vi "Add_spot_dialog.vi"(7 "Modify":bool, 8 "TransformedPt":bool, 9 "ArrayOfPointNames":string[](array[string]), 10 "CurrentSessionInformation_IN":T2={"CollectionOfPoints"=[{"MetaDataFile"=path "", "X"=0.0, "Y"=0.0, "Z"=0.0, "Group"=0, "Rotation"=0.0, "Fiducial"=FALSE, "Magnification"=0.0, "Working_Distance"=0.0, "Notes"="", "Location Name/ID"="", "OtherRelatedDataFiles"=[], "Available"=FALSE}, {"MetaDataFile"=path "", "X"=0.0, "Y"=0.0, "Z"=0.0, "Group"=0, "Rotation"=0.0, "Fiducial"=FALSE, "Magnification"=0.0, "Working_Distance"=0.0, "Notes"="", "Location Name/ID"="", "OtherRelatedDataFiles"=[], "Available"=FALSE}, {"MetaDataFile"=path "", "X"=0.0, "Y"=0.0, "Z"=0.0, "Group"=0, "Rotation"=0.0, "Fiducial"=FALSE, "Magnification"=0.0, "Working_Distance"=0.0, "Notes"="", "Location Name/ID"="", "OtherRelatedDataFiles"=[], "Available"=FALSE}, {"MetaDataFile"=path "", "X"=0.0, "Y"=0.0, "Z"=0.0, "Group"=0, "Rotation"=0.0, "Fiducial"=FALSE, "Magnification"=0.0, "Working_Distance"=0.0, "Notes"="", "Location Name/ID"="", "OtherRelatedDataFiles"=[], "Available"=FALSE}, {"MetaDataFile"=path "", "X"=0.0, "Y"=0.0, "Z"=0.0, "Group"=0, "Rotation"=0.0, "Fiducial"=FALSE, "Magnification"=0.0, "Working_Distance"=0.0, "Notes"="", "Location Name/ID"="", "OtherRelatedDataFiles"=[], "Available"=FALSE}, {"MetaDataFile"=path "", "X"=0.0, "Y"=0.0, "Z"=0.0, "Group"=0, "Rotation"=0.0, "Fiducial"=FALSE, "Magnification"=0.0, "Working_Distance"=0.0, "Notes"="", "Location Name/ID"="", "OtherRelatedDataFiles"=[], "Available"=FALSE}, {"MetaDataFile"=path "", "X"=0.0, "Y"=0.0, "Z"=0.0, "Group"=0, "Rotation"=0.0, "Fiducial"=FALSE, "Magnification"=0.0, "Working_Distance"=0.0, "Notes"="", "Location Name/ID"="", "OtherRelatedDataFiles"=[], "Available"=FALSE}], "Instrument"=enum."MXRD MFC", "CollectionFile"=path "/INL Macintosh/Users/timothymcjunkin/Desktop/Diffusion couple/MXRD 9-13-10/xrd_session_for_corrected.xml", "Session Name/ID"="xrd_test", "SessionNotes"="Sample moved to XRD"}, 11 "PointInformation_IN":T1) -> (0 "PointInformationOut":T1, 1 "CurrentSessionInformationOut":T2={"CollectionOfPoints"=[{"MetaDataFile"=path "", "X"=0.0, "Y"=0.0, "Z"=0.0, "Group"=0, "Rotation"=0.0, "Fiducial"=FALSE, "Magnification"=0.0, "Working_Distance"=0.0, "Notes"="", "Location Name/ID"="", "OtherRelatedDataFiles"=[], "Available"=FALSE}, {"MetaDataFile"=path "", "X"=0.0, "Y"=0.0, "Z"=0.0, "Group"=0, "Rotation"=0.0, "Fiducial"=FALSE, "Magnification"=0.0, "Working_Distance"=0.0, "Notes"="", "Location Name/ID"="", "OtherRelatedDataFiles"=[], "Available"=FALSE}, {"MetaDataFile"=path "", "X"=0.0, "Y"=0.0, "Z"=0.0, "Group"=0, "Rotation"=0.0, "Fiducial"=FALSE, "Magnification"=0.0, "Working_Distance"=0.0, "Notes"="", "Location Name/ID"="", "OtherRelatedDataFiles"=[], "Available"=FALSE}, {"MetaDataFile"=path "", "X"=0.0, "Y"=0.0, "Z"=0.0, "Group"=0, "Rotation"=0.0, "Fiducial"=FALSE, "Magnification"=0.0, "Working_Distance"=0.0, "Notes"="", "Location Name/ID"="", "OtherRelatedDataFiles"=[], "Available"=FALSE}, {"MetaDataFile"=path "", "X"=0.0, "Y"=0.0, "Z"=0.0, "Group"=0, "Rotation"=0.0, "Fiducial"=FALSE, "Magnification"=0.0, "Working_Distance"=0.0, "Notes"="", "Location Name/ID"="", "OtherRelatedDataFiles"=[], "Available"=FALSE}, {"MetaDataFile"=path "", "X"=0.0, "Y"=0.0, "Z"=0.0, "Group"=0, "Rotation"=0.0, "Fiducial"=FALSE, "Magnification"=0.0, "Working_Distance"=0.0, "Notes"="", "Location Name/ID"="", "OtherRelatedDataFiles"=[], "Available"=FALSE}, {"MetaDataFile"=path "", "X"=0.0, "Y"=0.0, "Z"=0.0, "Group"=0, "Rotation"=0.0, "Fiducial"=FALSE, "Magnification"=0.0, "Working_Distance"=0.0, "Notes"="", "Location Name/ID"="", "OtherRelatedDataFiles"=[], "Available"=FALSE}], "Instrument"=enum."MXRD MFC", "CollectionFile"=path "/INL Macintosh/Users/timothymcjunkin/Desktop/Diffusion couple/MXRD 9-13-10/xrd_session_for_corrected.xml", "Session Name/ID"="xrd_test", "SessionNotes"="Sample moved to XRD"}, 3 "Cancel_OUT":bool)   [LabVIEW 2011]
doc: "This VI or subroutine launches a dialog box that serves various very similar functions depending on the input values of two flags. The general purpose is to allow the user to input the coordinates for a fiducial or other point of interest. The dialog will accept input for default coordinates if the calling routine has that information. The inputs include Modify and TransformedPt flags and Current Session Information Input Point Information and ArrayOfPointNames. Outputs include Cancel, Current Session Information and Output Point Information.\n\nPressing any of the add modify spots buttons launches a multi-purpose dialog box which is reconfigured to parts of the dialog box the user interacts with in each mode. This effectively reuses a lot of code that would have needed to be duplicated for the different cases. In the process makes this one dialog box more complicated. This dialog also gets called after a spot from a previous session dialog box is completed. Two types of additions are possible without a calculation, one for a fiducial and one for a spot of interest that is not a fiducial. The modify version of this dialog box is simply supplied with the exiting information from a spot and allows the user to change the spot information. It may be called from the modify or the edit button on the sample information tab or the current session tab. The only difference is where the information comes from and goes to.\n\nThe dialog box uses the fiducial flag in the PositionInformation_IN structure to indicate to the dialog box that it is a fiducial. Under this case the fiducial selector graphic and radio buttons will be visible. The point name will be grayed out and disabled in this mode. When the user selects a radio button the name will auto-populate. \n\nThis dialog has features to assist the user:\n1. If the user enters a name or selects a fiducial that can be calculated the software will inform the user that coordinates are available to assist in the location of the point. The current version of the software auto populates these values whether or not the user has already started to enter coordinates. This is not optimal and a future release of the software should track whether the program last entered values or whether the user did to make a more appropriate decision about the substitution.\n2. If the user enters a name that matches a point previously entered in the current session the user will be warned of the conflict.\n\nThe user may press the cancel button at any time to discard the point being entered.\n\nBesides separate fiducial modes of operation the dialog box responds differently depending on two input flags:\n1. Modify: If modify flag is true different instructions appear in the dialog box. Warning message about a fiducial being named the same as a previous spot is disabled, the new information is substituted in to the array of points instead of appended, and action to make this point unique by adding a random number to the point name is disabled. \n2. TranformedPt: If this flag is set, the user receives additional prompts to drive the instrument to the transformed coordinates, questioned as to whether the spot is close enough, allows the user to fine tune or rename if the spot is not close enough, and disables the warnings about the spot existing in a previous session."
uses:
  cm2nm_coordinate_information_v2.ctl
  cm2nm_sample_set.ctl
  Instrument_type_enum_v2.ctl
  cm2nm_fiducial_selector.ctl
panel:
  in  "StageRotation":dbl
  in  "Allow_nonstandard_fids":bool
  out "error out 2":errorcluster
  in  "Cancel Button":bool
  out "Original_group":i32
  out "Instructions":string
  in  "Group Coding":i32
  out "MetaDataAvailable":bool caption="Is a Fiducial"
  out "error out":errorcluster
  in  "Notes:":string
  in  "Tab Control":T4(tab)
  in  "Fiducial Selector":T5
  in  "Get Coordinates from Meta File":bool
  in  "Move to next screen":bool
  in  "Point Name":string
  in  "Z-Position":dbl
  in  "Y-Position":dbl
  in  "X-Position":dbl
  in  "MetaDataFile":path
  in  "Fiducial?":bool
  in  "Add A Spot Related Data File":bool caption="Add Another File\nRelated to this Spot"
  in  "Goto Previous Screen":bool caption="Press to Move to \nPrevious Screen"
  in  "Press to goto final Screen":bool caption="Press to Move to Next\nInformation Screen"
  out "OtherRelatedDataFiles":T6(array[cluster])
  out "Review Point Information":T1
  in  "Go Back to Correct":bool
  in  "AddToDataBase":bool
  # "Enter or confirm the\nspot  name and positions\n\nIf Metafile is available \nselect it in the MetaDatafile\nField and click Use MetaFile\nto extract MetaData\nFrom the file."
  # "This form allows you\nto add any number of\nfiles related to this\nspot on the sample.\nFor example spectra\nfiles or images other\nthan the file \ncontaining meta data."
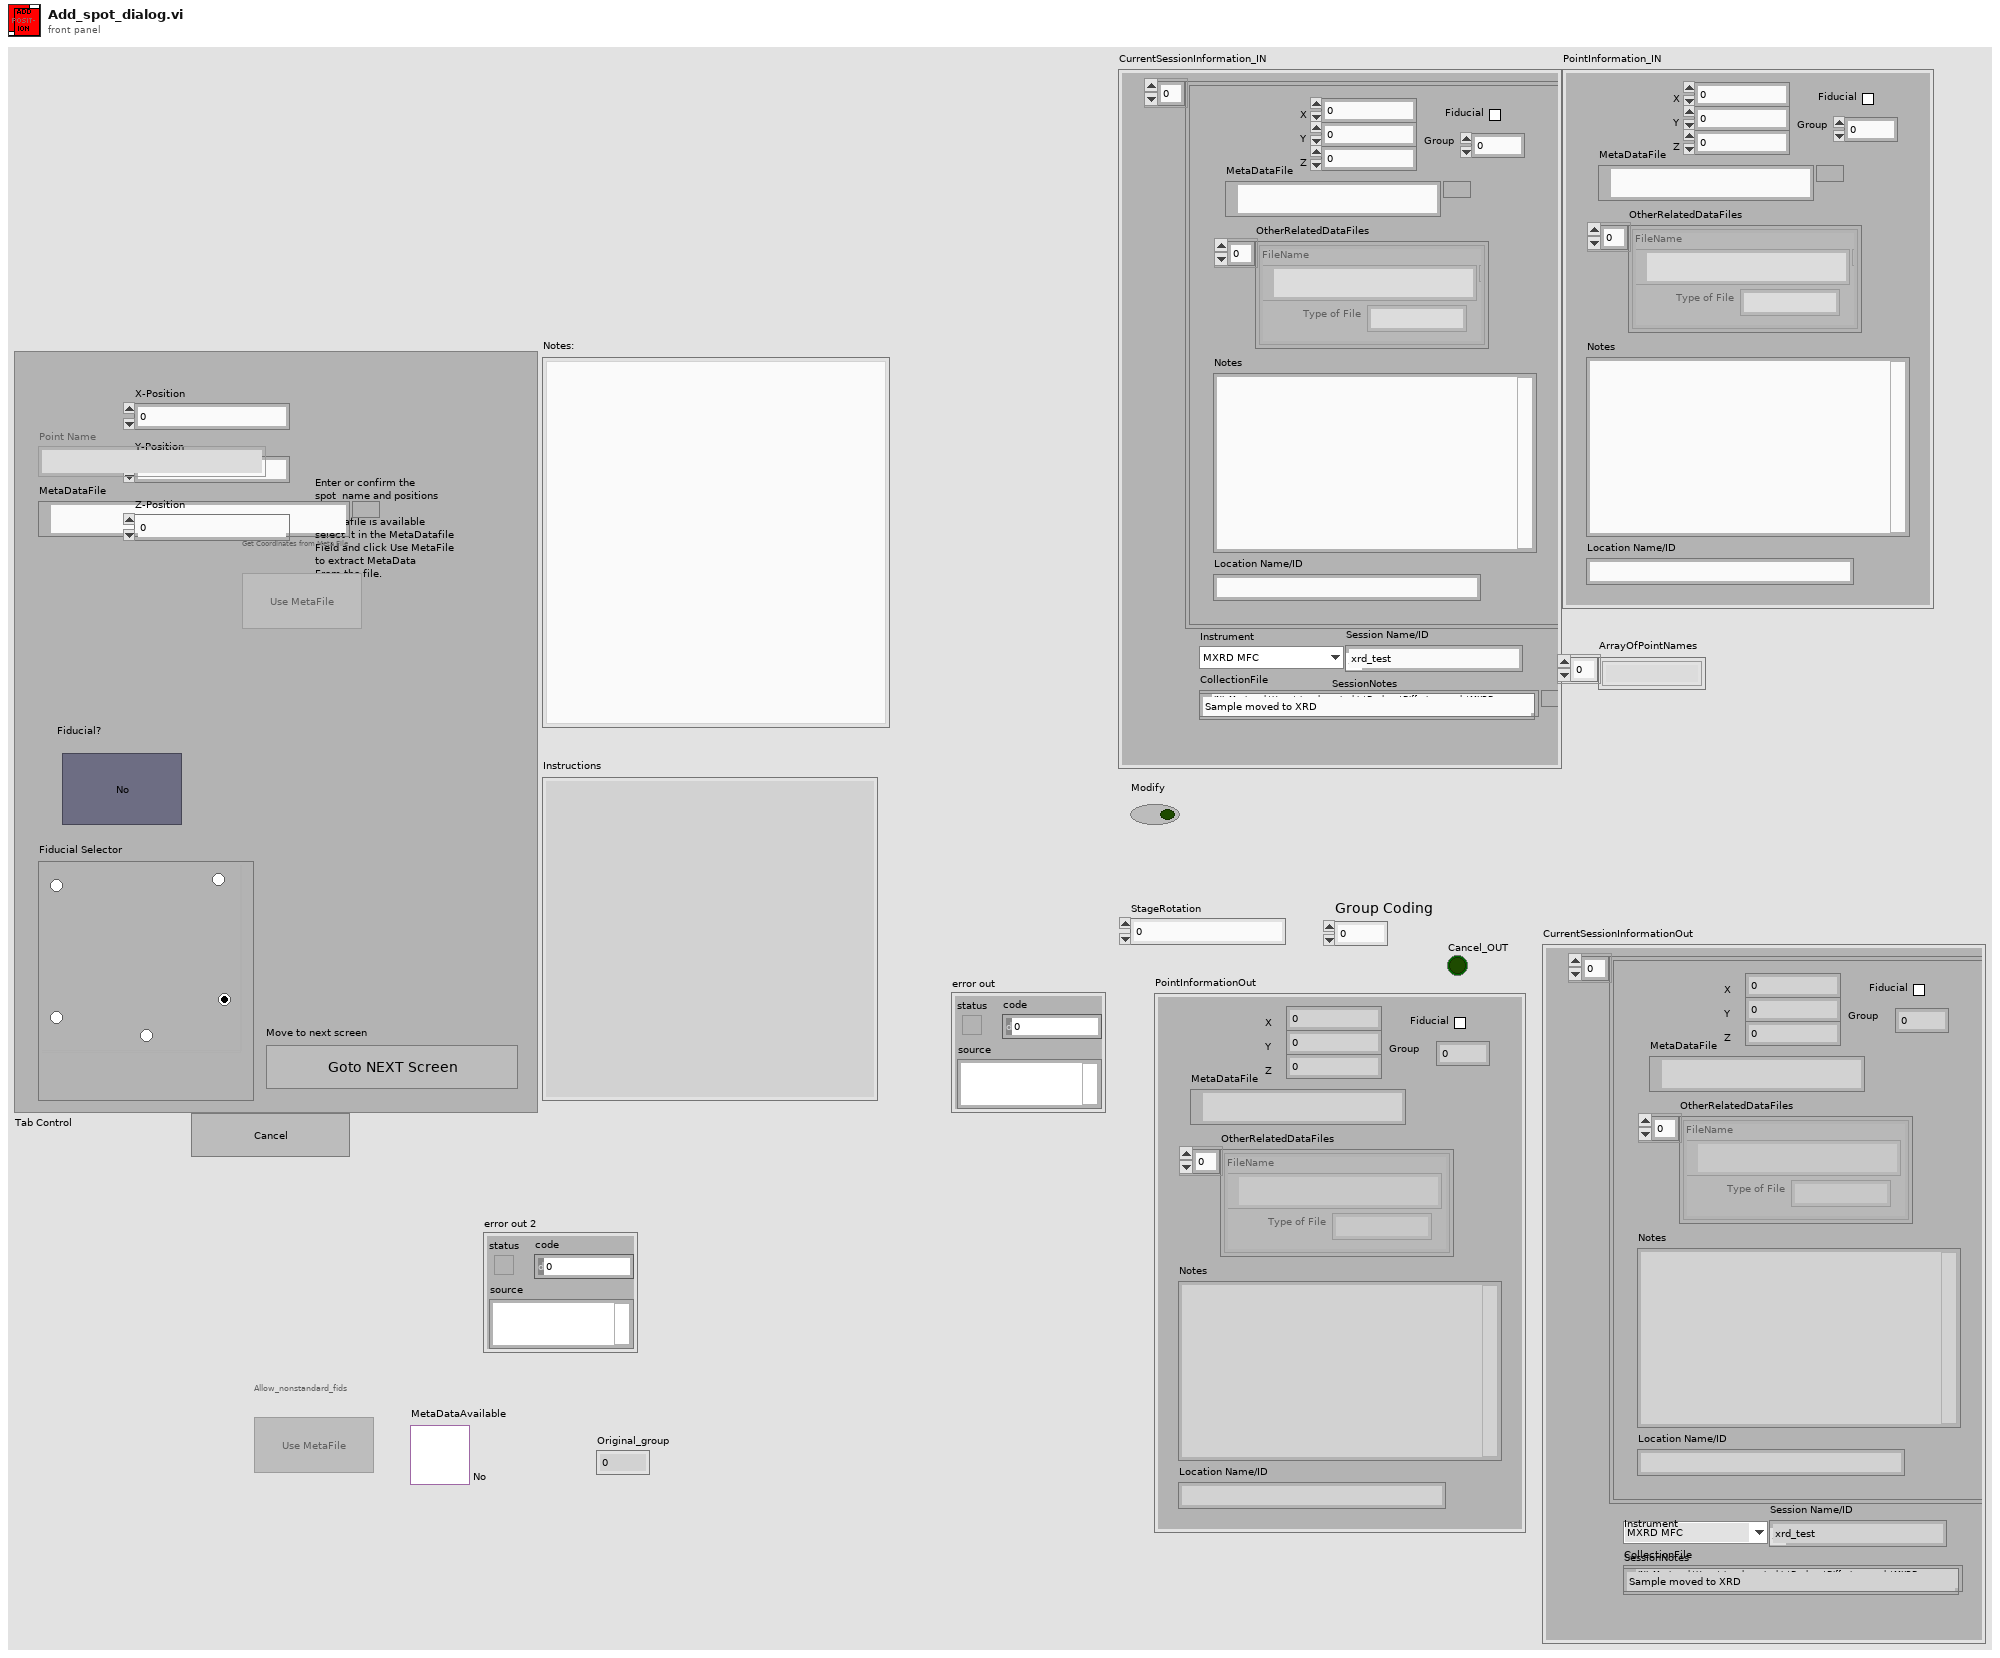
[diagram p1: front panel]
types:
  T1 = typedef "cm2nm_coordinate_information_v2.ctl" = cluster{"MetaDataFile":path, "X":dbl, "Y":dbl, "Z":dbl, "Group":i32, "Rotation":dbl[unit], "Fiducial":bool, "Magnification":dbl, "Working_Distance":dbl, "Notes":string, "Location Name/ID":string, "OtherRelatedDataFiles":cluster{"Type of File":string, "FileName":path}[], "Available":bool}
  T2 = typedef "cm2nm_sample_set.ctl" = cluster{"CollectionOfPoints":T1[], "Instrument":T3, "CollectionFile":path, "Session Name/ID":string, "SessionNotes":string}
  T3 = typedef "Instrument_type_enum_v2.ctl" = enum16{"Unknown", "Philips FEI SEM IRC", "JEOL 7000F EML_MFC", "MXRD MFC", "JEOL_EPMA"}
  T4 = enum32{"Name and Postions", "ExtraDataFiles", "SpotSummary"}
  T5 = typedef "cm2nm_fiducial_selector.ctl" = enum32{"Fiducial 1", "Fiducial 2", "Fiducial 3", "Fiducial 4", "Fiducial 5", "Other/NonStandard"}
  T6 = cluster{"Type of File":string, "FileName":path}[]
  T7 = enum8{"Enabled", "Disabled", "Disabled and Grayed Out"}
  T8 = enum32{"Name and Postions", "ExtraDataFiles", "SpotSummary", "Inputs"}
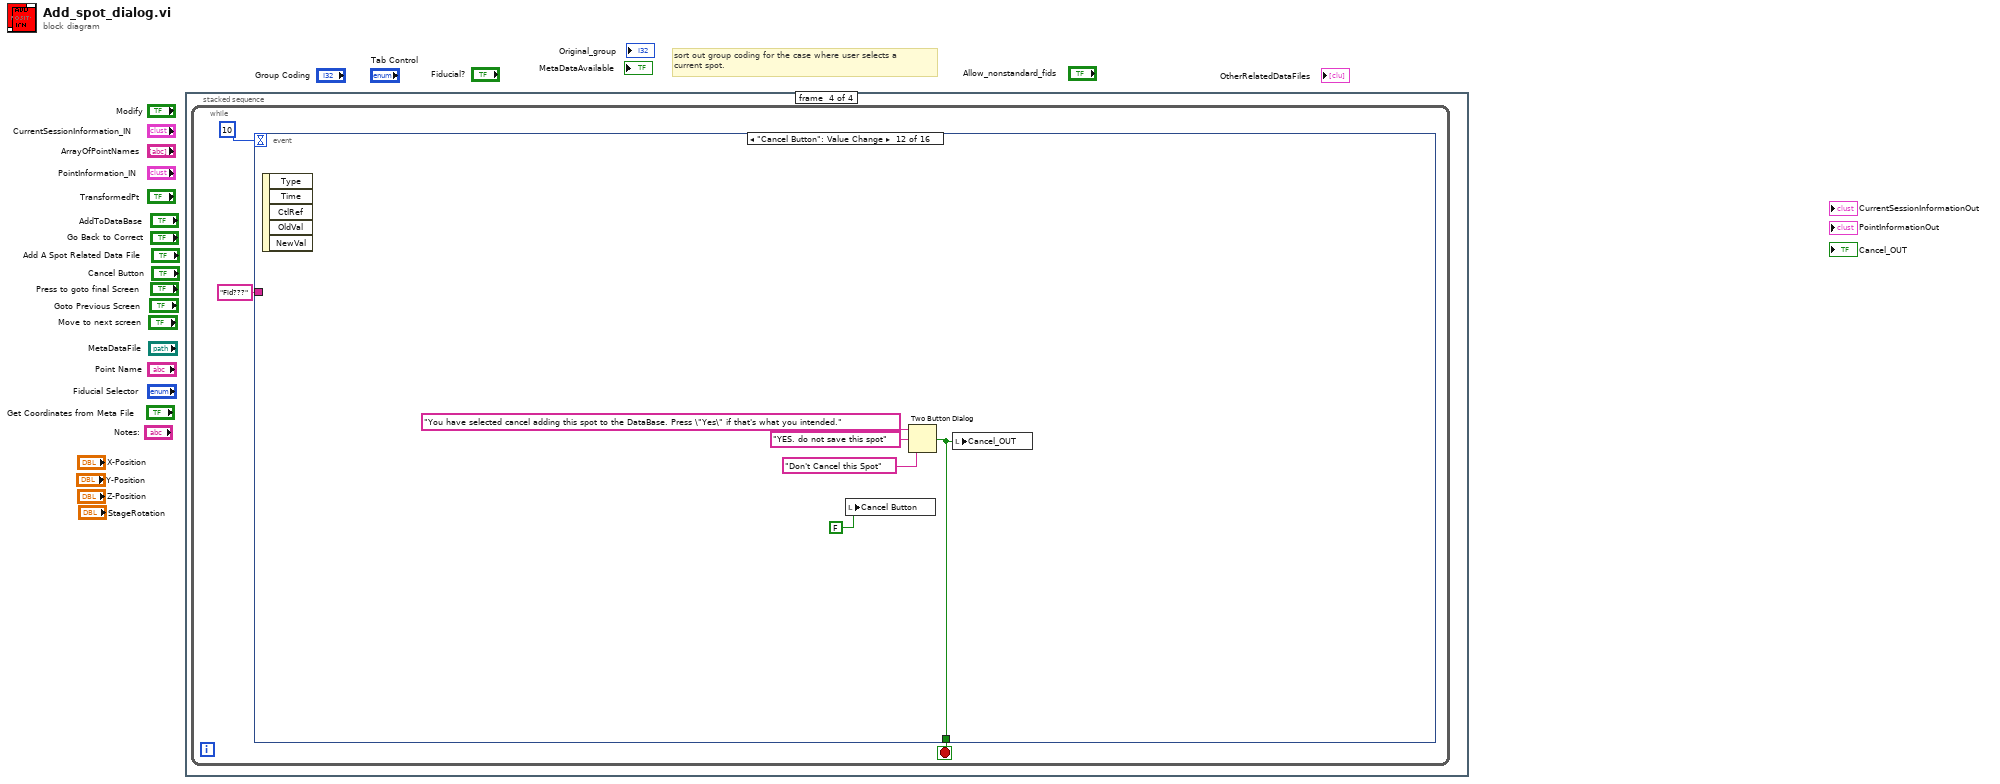
[diagram p0: block diagram]
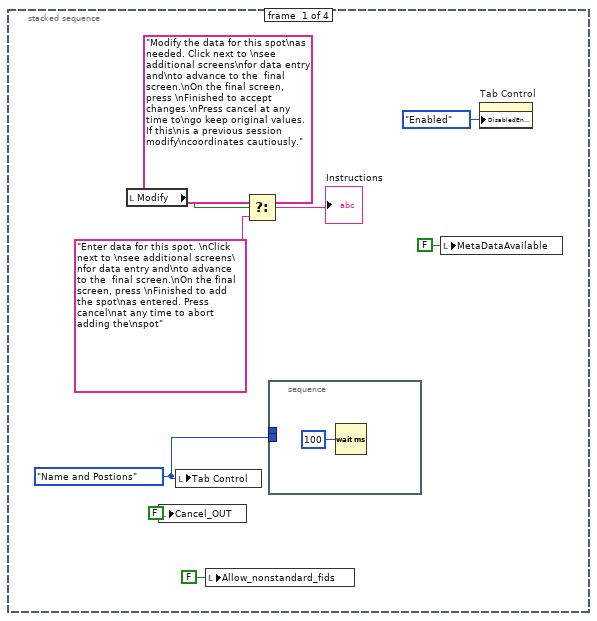
[diagram p2: hidden frame]
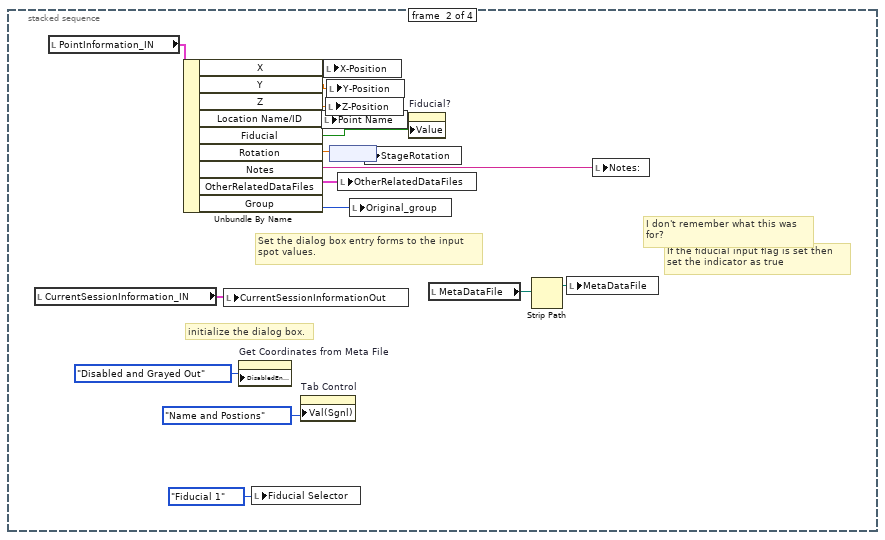
[diagram p3: hidden frame]
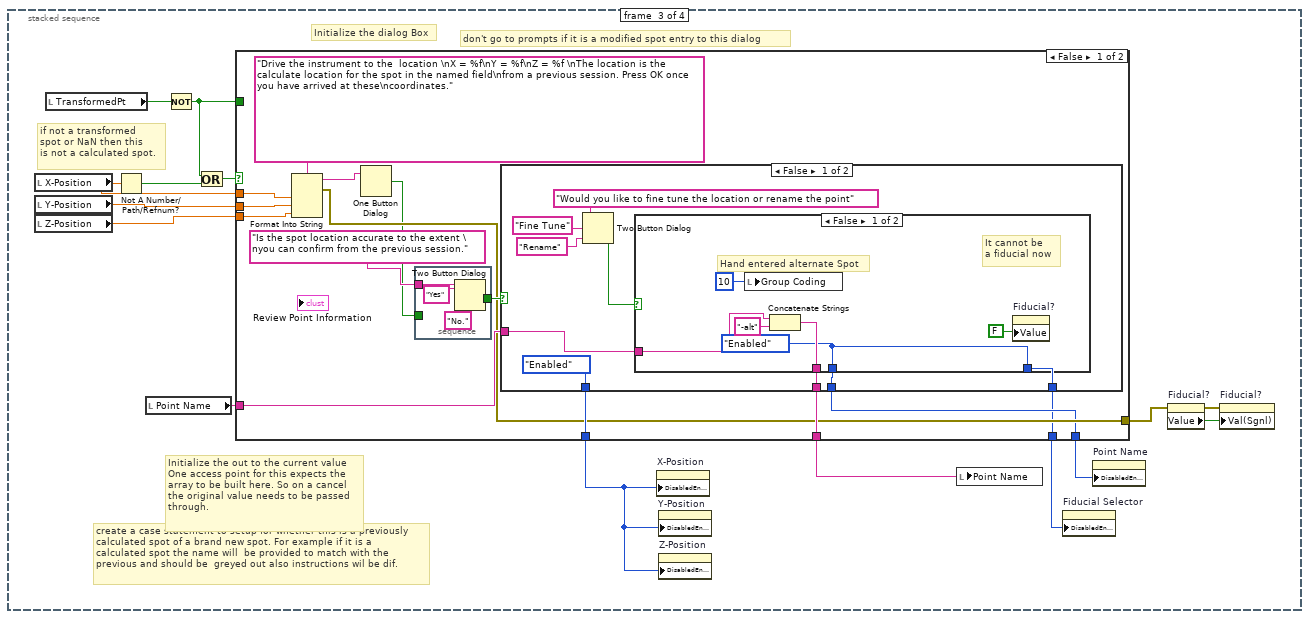
[diagram p4: hidden frame]
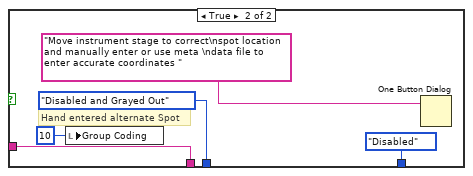
[diagram p5: hidden frame]
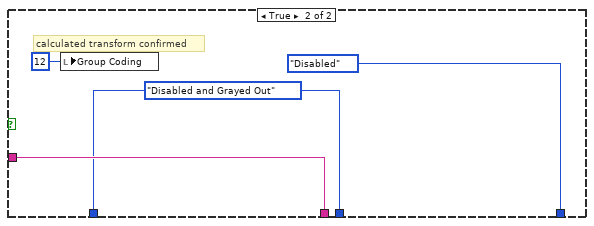
[diagram p6: hidden frame]
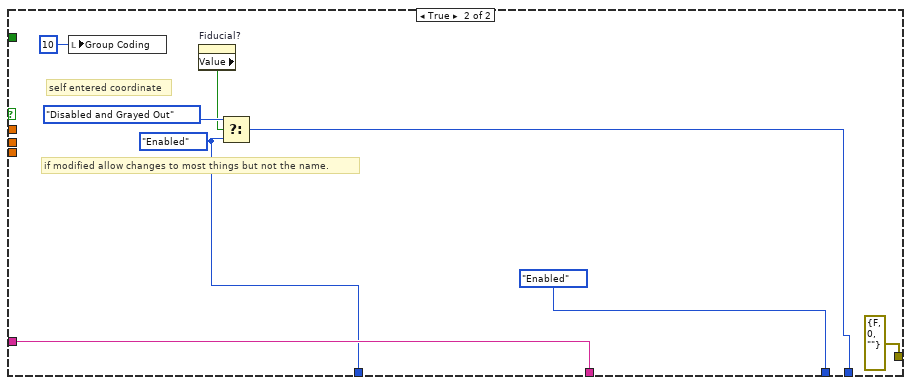
[diagram p7: hidden frame]
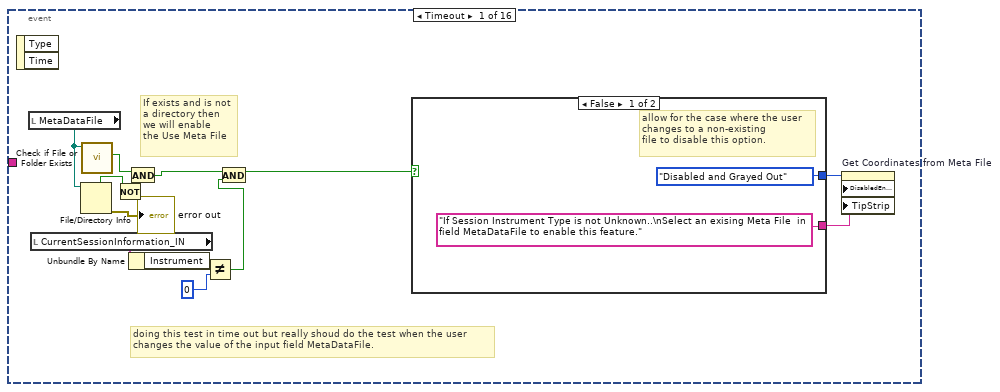
[diagram p8: hidden frame]
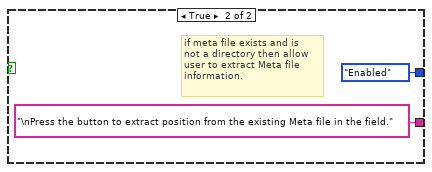
[diagram p9: hidden frame]
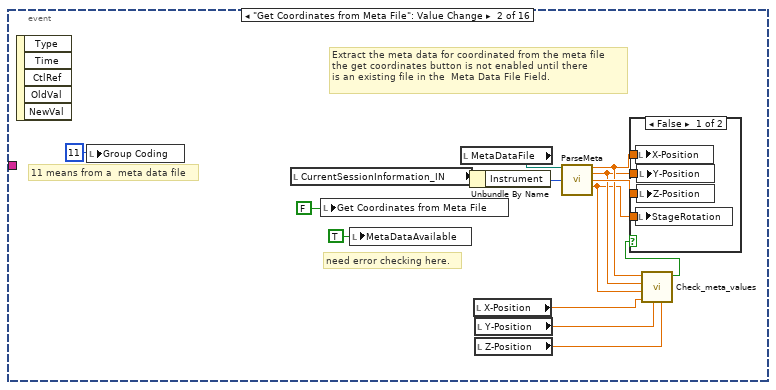
[diagram p10: hidden frame]
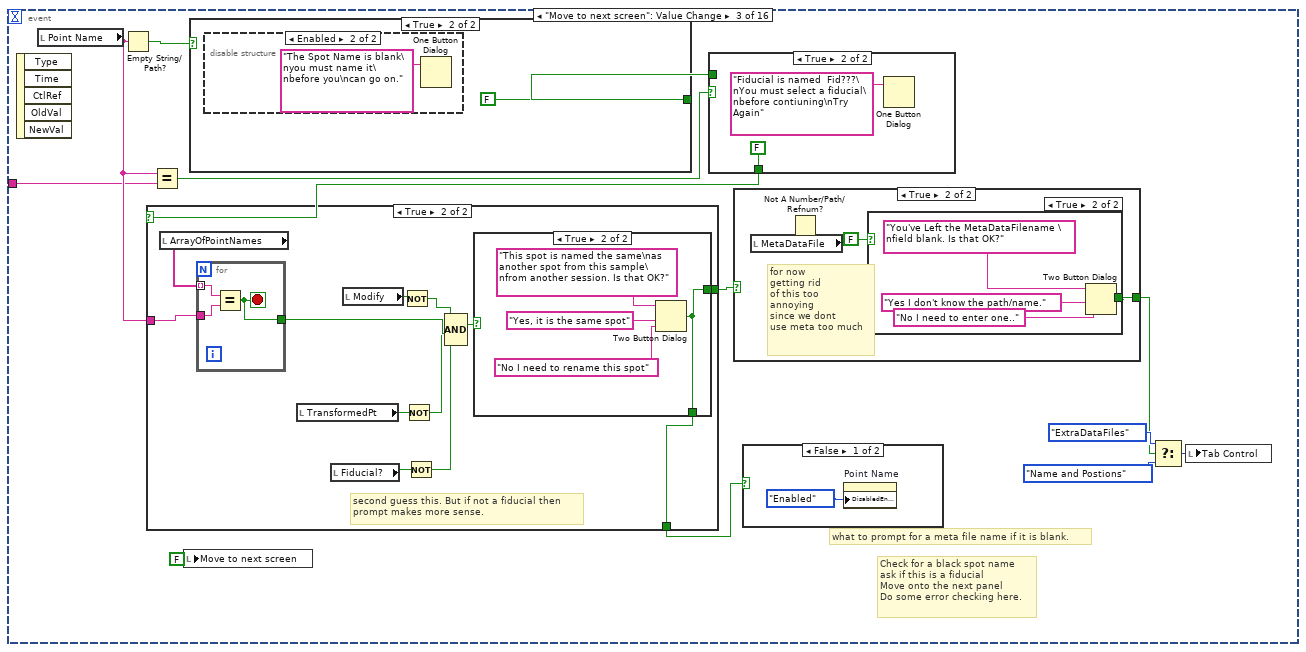
[diagram p12: hidden frame]
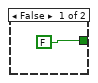
[diagram p15: hidden frame]
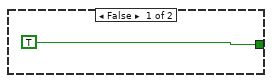
[diagram p16: hidden frame]
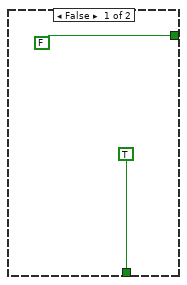
[diagram p17: hidden frame]
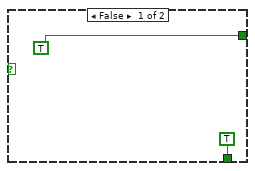
[diagram p18: hidden frame]
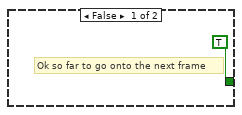
[diagram p19: hidden frame]
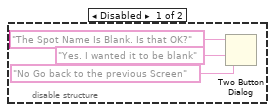
[diagram p20: hidden frame]
diagram:
  # "sort out group coding for the case where user selects a\ncurrent spot."
  n1 = stacked-sequence {
    frame #0 {
      w5 = T8."Name and Postions" ("Tab Control")
      n2 = local read "Modify"() -> (w6:bool)
      n3 = local write "Cancel_OUT"(FALSE ("Cancel")) -> ()
      n4 = local write "Tab Control"(w5) -> ()
      n5 = local write "Allow_nonstandard_fids"(FALSE ("Allow_nonstandard_fids")) -> ()
      n6 = Select(t="Modify the data for this spot\nas needed. Click next to \nsee additional screens\nfor data entry and\nto advance to the  final screen.\nOn the final screen, press \nFinished to accept changes.\nPress cancel at any time to\ngo keep original values. If this\nis a previous session modify\ncoordinates cautiously." ("Instructions"), s=w6, f="Enter data for this spot. \nClick next to \nsee additional screens\nfor data entry and\nto advance to the  final screen.\nOn the final screen, press \nFinished to add the spot\nas entered. Press cancel\nat any time to abort adding the\nspot" ("Instructions")) -> (s? t:f=→"Instructions":string)
      n7 = stacked-sequence {
        tunnel: [w10] -> _
        tunnel: w5 -> [w10]
        frame #0 {
          n8 = Wait (ms)(milliseconds to wait=u32 100) -> ()  [unwired: 1 out]
        }
      }
      n9 = local write "MetaDataAvailable"(FALSE ("MetaDataAvailable")) -> ()
      n10 = property on="Tab Control" class="TabCtl (strict)"("DisabledEnum"=T7."Enabled" ("Disabled")) -> ()  [unwired: 2 in, 2 out]
    }
    frame #1 {
      # "initialize the dialog box."
      # "I don't remember what this was\nfor?"
      # "If the fiducial input flag is set then \nset the indicator as true"
      # "Set the dialog box entry forms to the input\nspot values."
      n11 = local read "CurrentSessionInformation_IN"() -> (w19:T2)
      n12 = local read "PointInformation_IN"() -> (w28:T1)
      n13 = Unbundle By Name(w28) -> ("X"=w20:dbl, "Y"=w27:dbl, "Z"=w25:dbl, "Location Name/ID"=w26:string, "Fiducial"=w14:bool, "Rotation"=w24:dbl[unit], "Notes"=w22:string, "OtherRelatedDataFiles"=w21:T6, "Group"=w12:i32)
      n14 = local write "CurrentSessionInformationOut"(w19) -> ()
      n15 = property on="Get Coordinates from Meta File" class="Bool (strict)"("DisabledEnum"=T7."Disabled and Grayed Out" ("Disabled")) -> ()  [unwired: 2 in, 2 out]
      n16 = local write "Fiducial Selector"(cm2nm_fiducial_selector."Fiducial 1" ("Fiducial Selector")) -> ()
      n17 = property on="Tab Control" class="TabCtl (strict)"("Val(Sgnl)"=T8."Name and Postions" ("Tab Control")) -> ()  [unwired: 2 in, 2 out]
      n18 = local write "Point Name"(w26) -> ()
      n19 = local write "X-Position"(w20) -> ()
      n20 = local write "Z-Position"(w25) -> ()
      n21 = local write "Y-Position"(w27) -> ()
      n22 = node(w24) -> (w23:dbl)
      n23 = local write "OtherRelatedDataFiles"(w21) -> ()
      n24 = local write "Original_group"(w12) -> ()
      n25 = local write "StageRotation"(w23) -> ()
      n26 = property on="Fiducial?" class="Bool (strict)"("Value"=w14) -> ()  [unwired: 2 in, 2 out]
      n27 = local read "MetaDataFile"() -> (w16:path)
      n28 = Strip Path(path=w16) -> (stripped path=w15:path)  [unwired: 1 out]
      n29 = local write "MetaDataFile"(w15) -> ()
      n30 = local write "Notes:"(w22) -> ()
    }
    frame #2 {
      # "if not a transformed\nspot or NaN then this\nis not a calculated spot."
      # "don't go to prompts if it is a modified spot entry to this dialog"
      # "Initialize the out to the current value\nOne access point for this expects the\narray to be built here. So on a cancel\nthe original value needs to be passed\nthrough."
      # "Initialize the dialog Box"
      # "create a case statement to setup for whether this is a previously\ncalculated spot of a brand new spot. For example if it is a\ncalculated spot the name will  be provided to match with the \nprevious and should be  greyed out also instructions wil be dif."
      n31 = local read "X-Position"() -> (w38:dbl)
      n32 = local read "Y-Position"() -> (w40:dbl)
      n33 = local read "Z-Position"() -> (w39:dbl)
      n34 = local read "TransformedPt"() -> (w31:bool)
      n35 = Not A Number/Path/Refnum?(number/path/refnum=w38) -> (NaN/Path/Refnum?=w36:bool)
      n36 = local read "Point Name"() -> (w37:string)
      n37 = Not(x=w31) -> (.not. x?=w35:bool)
      n38 = Or(x=w35, y=w36) -> (x .or. y?=w41:bool)
      n39 = case shown="False" w41 {
        tunnel: [w50 w89] -> w43
        tunnel: w38 -> [w56 _]
        tunnel: w40 -> [w55 _]
        tunnel: [w45 w90] -> w30
        tunnel: w37 -> [w49 w93]
        tunnel: [w48 w93] -> w42
        tunnel: w39 -> [w52 _]
        tunnel: w35 -> [_ _]
        tunnel: [w47 errorcluster {"status"=FALSE, "code"=0, "source"=""} ("error IO")] -> w33
        tunnel: [w44 T7."Enabled" ("Disabled")] -> w29
        frame False {
          n40 = Format Into String(format string="Drive the instrument to the  location \nX = %f\nY = %f\nZ = %f \nThe location is the calculate location for the spot in the named field\nfrom a previous session. Press OK once you have arrived at these\ncoordinates.", w56, w55, w52) -> (resulting string=w54:string, error out=w47:errorcluster)  [unwired: 2 in]
          n41 = One Button Dialog ("Drive to the Calculated Coordinates")(message=w54) -> (true=w46:bool)  [unwired: 1 in]
          n42 = stacked-sequence {
            tunnel: "Is the spot location accurate to the extent \nyou can confirm from the previous session." -> [w61]
            tunnel: [w58] -> w51
            tunnel: w46 -> [_]
            frame #0 {
              n43 = Two Button Dialog(message=w61, 1:"No." ("F button name (\"Cancel\")"), 2:"Yes" ("T button name (\"OK\")")) -> (T button?=w58:bool)
            }
          }
          n44 = case shown="False" w51 {
            tunnel: [T7."Enabled" ("Disabled") w84] -> w50
            tunnel: w49 -> [w65 w85]
            tunnel: [w64 w85] -> w48
            tunnel: [w63 w84] -> w45
            tunnel: [w62 T7."Disabled" ("Disabled")] -> w44
            frame False {
              n45 = Two Button Dialog(message="Would you like to fine tune the location or rename the point", 1:"Rename" ("F button name (\"Cancel\")"), 2:"Fine Tune" ("T button name (\"OK\")")) -> (T button?=w66:bool)
              n46 = case shown="False" w66 {
                tunnel: w65 -> [w75 w81]
                tunnel: [w74 w81] -> w64
                tunnel: [w71 T7."Disabled and Grayed Out" ("Disabled")] -> w63
                tunnel: [w71 T7."Disabled" ("Disabled")] -> w62
                frame False {
                  w71 = T7."Enabled" ("Disabled")
                  # "It cannot be\na fiducial now"
                  # "Hand entered alternate Spot"
                  n47 = local write "Group Coding"(10 ("Group Coding")) -> ()
                  n48 = Concatenate Strings(w75, "-alt" ("string")) -> (w74:string)
                  n49 = property on="Fiducial?" class="Bool (strict)"("Value"=FALSE ("Fiducial?")) -> ()  [unwired: 2 in, 2 out]
                }
                frame True {
                  # "Hand entered alternate Spot"
                  n50 = local write "Group Coding"(10 ("Group Coding")) -> ()
                  n51 = One Button Dialog ("Drive to the Calculated Coordinates")(message="Move instrument stage to correct\nspot location and manually enter or use meta \ndata file to enter accurate coordinates ") -> ()  [unwired: 1 in, 1 out]
                }
              }
            }
            frame True {
              w84 = T7."Disabled and Grayed Out" ("Disabled")
              # "calculated transform confirmed"
              n52 = local write "Group Coding"(12 ("Group Coding")) -> ()
            }
          }
        }
        frame True {
          w89 = T7."Enabled" ("Disabled")
          # "if modified allow changes to most things but not the name."
          # "self entered coordinate"
          n53 = local write "Group Coding"(10 ("Group Coding")) -> ()
          n54 = property on="Fiducial?" class="Bool (strict)"() -> ("Value"=w87:bool)  [unwired: 2 in, 2 out]
          n55 = Select(t=T7."Disabled and Grayed Out" ("Disabled"), s=w87, f=w89) -> (s? t:f=w90:T7)
        }
      }
      n56 = property on="X-Position" class="DigNum (strict)"("DisabledEnum"=w43) -> ()  [unwired: 2 in, 2 out]
      n57 = property on="Y-Position" class="DigNum (strict)"("DisabledEnum"=w43) -> ()  [unwired: 2 in, 2 out]
      n58 = property on="Z-Position" class="DigNum (strict)"("DisabledEnum"=w43) -> ()  [unwired: 2 in, 2 out]
      n59 = local write "Point Name"(w42) -> ()
      n60 = property on="Fiducial Selector" class="RadioBtnsControl (strict)"("DisabledEnum"=w29) -> ()  [unwired: 2 in, 2 out]
      n61 = property on="Point Name" class="Str"("DisabledEnum"=w30) -> ()  [unwired: 2 in, 2 out]
      n62 = property on="Fiducial?" class="Bool (strict)"(error in=w33) -> (error out=w34:errorcluster, "Value"=w32:bool)  [unwired: 1 in, 1 out]
      n63 = property on="Fiducial?" class="Bool (strict)"(error in=w34, "Val(Sgnl)"=w32) -> ()  [unwired: 1 in, 2 out]
    }
    frame #3 {
      n64 = while {
        stop <- w95 stop-if-true
        n65 = event shown="[11] \"Cancel Button\": Value Change" {
          selector: _ -> [_ _ _ _ _ _ _ _ _ _ _ _ _ _ _ _]
          dyn-events: _ -> [_ _ _ _ _ _ _ _ _ _ _ _ _ _ _ _]
          timeout: 10 -> [_ _ _ _ _ _ _ _ _ _ _ _ _ _ _ _]
          tunnel: [_ _ _ _ _ TRUE ("T button?") w257 _ _ _ _ w376 _ _ _ _] -> w95
          tunnel: "Fid???" ("Value (Signaling)") -> [_ _ w136 _ w213 _ _ _ _ _ _ _ _ _ _ _]
          event Timeout {
            # "doing this test in time out but really shoud do the test when the user\nchanges the value of the input field MetaDataFile."
            # "If exists and is not\na directory then\nwe will enable \nthe Use Meta File"
            n66 = event-data() -> ()  [unwired: 1 in, 2 out]
            n67 = local read "MetaDataFile"() -> (w102:path)
            n68 = local read "CurrentSessionInformation_IN"() -> (w101:T2)
            n69 = File/Directory Info(path=w102) -> (directory=w109:bool, error out=→"error out":errorcluster)  [unwired: 1 in, 5 out]
            n70 = call <vilib>:"Check if File or Folder Exists.vi"("path"=w102) -> ("file or folder exists?"=w107:bool)  [unwired: 8 in, 2 out]
            n71 = Not(x=w109) -> (.not. x?=w108:bool)
            n72 = And(x=w107, y=w108) -> (x .and. y?=w103:bool)
            n73 = Unbundle By Name(w101) -> ("Instrument"=w100:T3)
            n74 = Not Equal?(x=w100, y=u16 0) -> (x != y?=w97:bool)
            n75 = And(x=w103, y=w97) -> (x .and. y?=w98:bool)
            n76 = case shown="False" w98 {
              tunnel: [T7."Disabled and Grayed Out" ("Disabled") T7."Enabled" ("Disabled")] -> w105
              tunnel: ["If Session Instrument Type is not Unknown..\nSelect an exising Meta File  in field MetaDataFile to enable this feature." ("Tip Strip") "\nPress the button to extract position from the existing Meta file in the field." ("Tip Strip")] -> w104
              frame False {
                # "allow for the case where the user\nchanges to a non-existing\nfile to disable this option."
              }
              frame True {
                # "if meta file exists and is\nnot a directory then allow \nuser to extract Meta file \ninformation."
              }
            }
            n77 = property on="Get Coordinates from Meta File" class="Bool (strict)"("DisabledEnum"=w105, "TipStrip"=w104) -> ()  [unwired: 2 in, 2 out]
          }
          event "Get Coordinates from Meta File": Value Change {
            # "11 means from a  meta data file"
            # "need error checking here."
            # "Extract the meta data for coordinated from the meta file\nthe get coordinates button is not enabled until there\nis an existing file in the  Meta Data File Field."
            n78 = event-data() -> ()  [unwired: 1 in, 5 out]
            n79 = local write "Group Coding"(11 ("Group Coding")) -> ()
            n80 = local read "CurrentSessionInformation_IN"() -> (w122:T2)
            n81 = local write "Get Coordinates from Meta File"(FALSE ("Get Coords")) -> ()
            n82 = local write "MetaDataAvailable"(TRUE ("MetaDataAvailable")) -> ()
            n83 = local read "MetaDataFile"() -> (w126:path)
            n84 = Unbundle By Name(w122) -> ("Instrument"=w125:T3)
            n85 = local read "X-Position"() -> (w117:dbl)
            n86 = local read "Y-Position"() -> (w116:dbl)
            n87 = local read "Z-Position"() -> (w115:dbl)
            n88 = call "ParseMeta.vi"("Path"=w126, "Instrument"=w125) -> ("X-stage (um)"=w120:dbl, "Y-stage (um)"=w119:dbl, "Z-stage (um)"=w124:dbl, "R-stage (deg)"=w118:dbl)  [unwired: 1 in, 9 out]
            n89 = call "Check_meta_values.vi"("Z-Position"=w115, "Y-Position"=w116, "X-Position"=w117, "Z-Position_M"=w118, "Y-Position_M"=w119, "X-Position_M"=w120) -> ("Cancelled?"=w114:bool)  [unwired: 5 in]
            n90 = case shown="False" w114 {
              tunnel: w124 -> [w131 _]
              tunnel: w120 -> [w130 _]
              tunnel: w119 -> [w129 _]
              tunnel: w118 -> [w128 _]
              frame False {
                n91 = local write "X-Position"(w130) -> ()
                n92 = local write "StageRotation"(w128) -> ()
                n93 = local write "Y-Position"(w129) -> ()
                n94 = local write "Z-Position"(w131) -> ()
              }
              frame True {
              }
            }
          }
          event "Move to next screen": Value Change {
            # "what to prompt for a meta file name if it is blank."
            # "Check for a black spot name\nask if this is a fiducial\nMove onto the next panel\nDo some error checking here."
            n95 = event-data() -> ()  [unwired: 1 in, 5 out]
            n96 = local read "Point Name"() -> (w137:string)
            n97 = Empty String/Path?(string/path=w137) -> (empty?=w143:bool)
            n98 = Equal?(x=w137, y=w136) -> (x = y?=w135:bool)
            n99 = local write "Move to next screen"(FALSE ("Press to Move to Next\nInformation Screen")) -> ()
            n100 = case shown="True" w143 {
              tunnel: [TRUE ("T button?") FALSE ("T button?")] -> w134
              frame False {
                # "Ok so far to go onto the next frame"
              }
              frame True {
                n101 = disable-structure shown="Enabled" {
                  frame Disabled {
                    n102 = Two Button Dialog(message="The Spot Name Is Blank. Is that OK?", 1:"No Go back to the previous Screen" ("F button name (\"Cancel\")"), 2:"Yes. I wanted it to be blank" ("T button name (\"OK\")")) -> ()  [unwired: 1 out]
                  }
                  frame Enabled {
                    n103 = One Button Dialog(message="The Spot Name is blank\nyou must name it\nbefore you\ncan go on.") -> ()  [unwired: 1 in, 1 out]
                  }
                }
              }
            }
            n104 = case shown="True" w135 {
              tunnel: w134 -> [w145 _]
              tunnel: [w145 FALSE ("T button?")] -> w133
              frame False {
              }
              frame True {
                n105 = One Button Dialog(message="Fiducial is named  Fid???\nYou must select a fiducial\nbefore contiuning\nTry Again") -> ()  [unwired: 1 in, 1 out]
              }
            }
            n106 = case shown="True" w133 {
              tunnel: w137 -> [_ w170]
              tunnel: [FALSE ("T button?") w168] -> w142
              tunnel: [TRUE ("T button?") w167] -> w132
              frame False {
              }
              frame True {
                # "second guess this. But if not a fiducial then \nprompt makes more sense."
                n107 = local read "ArrayOfPointNames"() -> (w171:string[])
                n108 = for {
                  tunnel: w171 -> [w180] mode=indexing
                  tunnel: w170 -> [w179]
                  tunnel: [w178] -> w169
                  stop <- w178 stop-if-true
                  n109 = Equal?(x=w180, y=w179) -> (x = y?=w178:bool)
                }
                n110 = local read "TransformedPt"() -> (w160:bool)
                n111 = local read "Fiducial?"() -> (w162:bool)
                n112 = local read "Modify"() -> (w163:bool)
                n113 = Not(x=w163) -> (.not. x?=w164:bool)
                n114 = Not(x=w160) -> (.not. x?=w165:bool)
                n115 = Not(x=w162) -> (.not. x?=w161:bool)
                n116 = Compound Arithmetic op=AND(w164, w165, w169, w161) -> (w166:bool)
                n117 = case shown="True" w166 {
                  tunnel: [TRUE ("T button?") w174] -> w168
                  tunnel: [TRUE ("T button?") w174] -> w167
                  frame False {
                  }
                  frame True {
                    n118 = Two Button Dialog(message="This spot is named the same\nas another spot from this sample\nfrom another session. Is that OK?", 1:"No I need to rename this spot" ("F button name (\"Cancel\")"), 2:"Yes, it is the same spot" ("T button name (\"OK\")")) -> (T button?=w174:bool)
                  }
                }
              }
            }
            n119 = case shown="True" w142 {
              tunnel: [FALSE ("T button?") w151] -> w138
              frame False {
              }
              frame True {
                # "for now\ngetting rid \nof this too\nannoying\nsince we dont\nuse meta too much"
                n120 = local read "MetaDataFile"() -> (w152:path)
                n121 = Not A Number/Path/Refnum?(number/path/refnum=w152) -> ()  [unwired: 1 out]
                n122 = case shown="True" FALSE {
                  tunnel: [TRUE ("T button?") w154] -> w151
                  frame False {
                  }
                  frame True {
                    n123 = Two Button Dialog(message="You've Left the MetaDataFilename \nfield blank. Is that OK?", 1:"No I need to enter one.." ("F button name (\"Cancel\")"), 2:"Yes I don't know the path/name." ("T button name (\"OK\")")) -> (T button?=w154:bool)
                  }
                }
              }
            }
            n124 = case shown="False" w132 {
              frame False {
                n125 = property on="Point Name" class="Str"("DisabledEnum"=T7."Enabled" ("Disabled")) -> ()  [unwired: 2 in, 2 out]
              }
              frame True {
              }
            }
            n126 = Select(t=T8."ExtraDataFiles" ("Tab Control"), s=w138, f=T8."Name and Postions" ("Tab Control")) -> (s? t:f=w141:T8)
            n127 = local write "Tab Control"(w141) -> ()
          }
          event "Fiducial?": Value Change {
            n128 = event-data() -> ("CtlRef"=w187:refnum<vi>, "OldVal"=w190:bool, "NewVal"=w189:bool)  [unwired: 1 in, 2 out]
            n129 = Not Equal?(x=w190, y=w189) -> (x != y?=w188:bool)
            n130 = case shown="False" w188 {
              tunnel: [TRUE ("T button?") w194] -> w191
              tunnel: w189 -> [_ w193]
              frame False {
              }
              frame True {
                n131 = Select(t="You have changed this\nspot to be a fiducial.\nIs this correct?" ("message"), s=w193, f="You have changed this\nspot to NOT be a fiducial.\nIs this correct?\nIf YES please check the verify the Spot Name." ("message")) -> (s? t:f=w197:string)
                n132 = Two Button Dialog(message=w197, 1:"No" ("F button name (\"Cancel\")"), 2:"Yes" ("T button name (\"OK\")")) -> (T button?=w194:bool)
              }
            }
            n133 = property on="Fiducial Selector" class="RadioBtnsControl (strict)"("Visible"=w189) -> ()  [unwired: 2 in, 2 out]
            n134 = case shown="True" w191 {
              tunnel: w187 -> [w202 _]
              tunnel: w190 -> [w201 _]
              tunnel: w189 -> [_ w203]
              frame False {
                n135 = property class="Bool (strict)"(reference=w202, "Value"=w201) -> ()  [unwired: 1 in, 2 out]
                n136 = property on="Point Name" class="Str"("DisabledEnum"=T7."Enabled" ("Disabled")) -> ()  [unwired: 2 in, 2 out]
              }
              frame True {
                # "This cause a blank fiducial name to\nbecome a non standard fiducial.\nWhich is ok."
                # "if fiducial make this visible"
                n137 = local read "PointInformation_IN"() -> (w204:T1)
                n138 = case shown="True" w203 {
                  frame False {
                  }
                  frame True {
                    n139 = local read "Point Name"() -> (w212:string)
                    n140 = Scan From String(format string="Fid%d", input string=w212, default 1=6 ("default value 1")) -> (error out=→"error out 2":errorcluster, output 1=w209:i32)  [unwired: 2 in, 2 out]
                    n141 = property on="Point Name" class="Str"("DisabledEnum"=T7."Disabled and Grayed Out" ("Disabled")) -> ()  [unwired: 2 in, 2 out]
                    n142 = Decrement(x=w209) -> (x-1=w208:i32)
                    n143 = property on="Fiducial Selector" class="RadioBtnsControl (strict)"("Val(Sgnl)"=w208) -> ()  [unwired: 2 in, 2 out]
                  }
                }
                n144 = Bundle By Name(cluster=w204, "Fiducial"=w203) -> (w205:T1)
                n145 = local write "Review Point Information"(w205) -> ()
              }
            }
          }
          event Value Change {
            n146 = event-data() -> ("NewVal"=w215:T5)  [unwired: 1 in, 4 out]
            n147 = Greater?(x=w215, y=cm2nm_fiducial_selector."Fiducial 5" ("Fiducial Selector")) -> (0:w217:bool)
            n148 = case shown="True" w217 {
              tunnel: w215 -> [w222 _]
              tunnel: [T7."Disabled and Grayed Out" ("Disabled") T7."Enabled" ("Disabled")] -> w214
              tunnel: w213 -> [_ w223]
              frame False {
                # "signal value change to check\nthe fiducial for duplicates."
                # "Auto assign the fiducial name."
                n149 = Increment(x=w222) -> (x+1=w221:T5)
                n150 = Format Into String(format string="Fid%d", w221) -> (resulting string=w218:string)  [unwired: 2 in, 1 out]
                n151 = property on="Point Name" class="Str"("Val(Sgnl)"=w218) -> ()  [unwired: 2 in, 2 out]
              }
              frame True {
                n152 = property on="Point Name" class="Str"("Val(Sgnl)"=w223) -> ()  [unwired: 2 in, 2 out]
                n153 = disable-structure shown="Disabled" {
                  frame Disabled {
                    n154 = One Button Dialog(message="Current Spot Name is a for\na non-standard\nFiducial\nDouble check\nthe Spot Name") -> ()  [unwired: 1 in, 1 out]
                  }
                  frame Enabled {
                  }
                }
              }
            }
            n155 = property on="Point Name" class="Str"("DisabledEnum"=w214) -> ()  [unwired: 2 in, 2 out]
          }
          event "AddToDataBase": Value Change {
            # "Add it to this array"
            n156 = event-data() -> ()  [unwired: 1 in, 5 out]
            n157 = local read "Review Point Information"() -> (w226:T1)
            n158 = local read "CurrentSessionInformation_IN"() -> (w228:T2)
            n159 = local write "PointInformationOut"(w226) -> ()
            n160 = Unbundle By Name(w228) -> ("CollectionOfPoints"=w231:T1[])
            n161 = local read "Modify"() -> (w229:bool)
            n162 = case shown="True" w229 {
              tunnel: w231 -> [w237 w241]
              tunnel: w226 -> [w236 w239]
              tunnel: [w235 w238] -> w230
              frame False {
                n163 = Build Array (concatenate)(w237, w236) -> (w235:T1[])
              }
              frame True {
                n164 = Unbundle By Name(w239) -> ("Location Name/ID"=w243:string)
                n165 = for {
                  tunnel: w241 -> [w255] mode=indexing
                  tunnel: w243 -> [w253]
                  tunnel: [w252] -> w242
                  tunnel: [w251] -> w240
                  i -> [w251]
                  stop <- w252 stop-if-true
                  n166 = Unbundle By Name(w255) -> ("Location Name/ID"=w254:string)
                  n167 = Equal?(x=w254, y=w253) -> (x = y?=w252:bool)
                }
                n168 = case shown="False" w242 {
                  tunnel: w241 -> [w246 w250]
                  tunnel: w240 -> [_ w249]
                  tunnel: w239 -> [w245 w248]
                  tunnel: [w244 w247] -> w238
                  frame False {
                    # "This means the name \nwas changed so add it"
                    n169 = Build Array (concatenate)(w246, w245) -> (w244:T1[])
                  }
                  frame True {
                    n170 = Replace Array Subset(array=w250, new element=w248, index=w249) -> (w247:T1[])
                  }
                }
              }
            }
            n171 = Bundle By Name(cluster=w228, "CollectionOfPoints"=w230) -> (w227:T2)
            n172 = stacked-sequence {
              tunnel: w227 -> [_]
              frame #0 {
                n173 = local write "Tab Control"(T4."Name and Postions" ("Tab Control")) -> ()
              }
            }
            n174 = local write "CurrentSessionInformationOut"(w227) -> ()
            n175 = local write "AddToDataBase"(FALSE ("AddToDataBase")) -> ()
          }
          event Panel Close? {
            # "Give user one more chance to not cancel."
            n176 = event-data() -> ()  [unwired: 1 in, 3 out]
            n177 = Two Button Dialog(message="You have selected cancel adding this spot to the DataBase. Press \"Yes\" if that's what you intended.", 1:"Don't Cancel this Spot" ("F button name (\"Cancel\")"), 2:"YES. do not save this spot" ("T button name (\"OK\")")) -> (T button?=w257:bool)
            n178 = local write "Cancel_OUT"(w257) -> ()
            n179 = local write "Cancel Button"(FALSE ("Cancel")) -> ()
            n180 = event-data("Discard?"=TRUE) -> ()  [unwired: 1 in, 1 out]
          }
          event "Goto Previous Screen": Value Change {
            n181 = event-data() -> ()  [unwired: 1 in, 5 out]
            n182 = local write "Goto Previous Screen"(FALSE ("Goto Previous Screen")) -> ()
            n183 = local write "Tab Control"(T8."Name and Postions" ("Tab Control")) -> ()
          }
          event "X-Position", "Y-Position", "Z-Position", "MetaDataFile": Value Change {
            # "If user changes any of these from the interface then the values did not come\nfrom the meta file and the indicator should be false."
            n184 = event-data() -> ("CtlRef"=w264:refnum<vi>, "OldVal"=w266:variant, "NewVal"=w265:variant)  [unwired: 1 in, 2 out]
            n185 = local read "Group Coding"() -> (w267:i32)
            n186 = case shown="11, 20" w267 {
              tunnel: w266 -> [_ _ w268]
              tunnel: w265 -> [_ _ _]
              tunnel: w264 -> [_ _ w269]
              frame 0, Default {
              }
              frame 10 {
                # "10 is ok  self entered no warning message for entering these values."
              }
              frame 11, 20 {
                # "coding from meta data file"
                n187 = Two Button Dialog(message="You have modified values\nread from the meta data\nfile or the meta data file name\n. Do you want to do \nthis?  ", 1:"No revert to the old meta data Value" ("F button name (\"Cancel\")"), 2:"Yes, keep the new values" ("T button name (\"OK\")")) -> (T button?=w270:bool)
                n188 = case shown="True" w270 {
                  tunnel: w269 -> [w274 _]
                  tunnel: w268 -> [w275 _]
                  frame False {
                    n189 = property class="Ctl"(reference=w274, "Value"=w275) -> ()  [unwired: 1 in, 2 out]
                  }
                  frame True {
                    # "change to 10 so the user\ncan modify as needed"
                    n190 = local write "Group Coding"(10 ("Group Coding")) -> ()
                  }
                }
              }
            }
          }
          event "X-Position", "Y-Position", "Z-Position": Mouse Enter {
            # "check for not a number. We do this here because the button may have been disabled\ndue to reselection of a repeated fiducial. User is required to touch one of the x/y/z\nfield to continue."
            n191 = event-data() -> ()  [unwired: 1 in, 3 out]
            n192 = local read "X-Position"() -> (w281:dbl)
            n193 = local read "Y-Position"() -> (w280:dbl)
            n194 = Not A Number/Path/Refnum?(number/path/refnum=w280) -> (NaN/Path/Refnum?=w278:bool)
            n195 = Not A Number/Path/Refnum?(number/path/refnum=w281) -> (NaN/Path/Refnum?=w279:bool)
            n196 = Or(x=w279, y=w278) -> (x .or. y?=w277:bool)
            n197 = case shown="True" w277 {
              tunnel: [T7."Enabled" ("Disabled") T7."Disabled and Grayed Out" ("Disabled")] -> w283
              tunnel: ["Click Next Once All Fields on this page are entered correctly" ("Tip Strip") "Enter valid numbers in X and Y Position to Continue" ("Tip Strip")] -> w282
              frame False {
              }
              frame True {
                # "allow for the case where the user\nchanges to a non-existing\nfile to disable this option."
              }
            }
            n198 = property on="Move to next screen" class="Bool (strict)"("DisabledEnum"=w283, "TipStrip"=w282) -> ()  [unwired: 2 in, 2 out]
          }
          event "Point Name": Value Change {
            (unwired) "Warning:\nYou have entered "
            # "minus 1 means\nnew to this session"
            # "if changed name of a type 10"
            # "handle duplicate fiducial by warning user and replacing data if user continues."
            n199 = event-data() -> ("OldVal"=w297:string, "NewVal"=w288:string)  [unwired: 1 in, 3 out]
            n200 = local read "CurrentSessionInformation_IN"() -> (w295:T2)
            n201 = Unbundle By Name(w295) -> ("CollectionOfPoints"=w294:T1[])
            n202 = for {
              tunnel: w294 -> [w300] mode=indexing
              tunnel: w288 -> [w301]
              tunnel: [w298] -> _
              tunnel: [w299] -> w291
              tunnel: [w300] -> w293
              tunnel: [w298] -> w292
              stop <- w298 stop-if-true
              n203 = Unbundle By Name(w300) -> ("Location Name/ID"=w302:string, "Group"=w299:i32)
              n204 = Equal?(x=w301, y=w302) -> (x = y?=w298:bool)
            }
            n205 = Not Equal?(x=w297, y=w288) -> (x != y?=w296:bool)
            n206 = Select(t=w291, s=w292, f=-1) -> (s? t:f=w289:i32)
            n207 = case shown="20, Default" w289 {
              tunnel: w297 -> [w305 _ _]
              tunnel: w296 -> [w304 _ w335]
              tunnel: w293 -> [w303 _ w336]
              tunnel: w288 -> [_ _ w334]
              tunnel: w289 -> [_ _ w333]
              tunnel: w288 -> [_ w324 _]
              frame 20, Default {
                # "need to check for a duplicate and\nreplace with the value."
                n208 = case shown="True" w304 {
                  tunnel: w305 -> [_ w308]
                  tunnel: w303 -> [_ w307]
                  frame False {
                  }
                  frame True {
                    n209 = disable-structure shown="Disabled" {
                      frame Disabled {
                        n210 = Two Button Dialog(message="You have changed a spot name of a point.\nassociated with other points in\nthe data base.\nDid you mean to do this?", 1:"No. Revert to the old name." ("F button name (\"Cancel\")"), 2:"Yes." ("T button name (\"OK\")")) -> ()  [unwired: 1 out]
                      }
                      frame Enabled {
                      }
                    }
                    n211 = case shown="False" FALSE {
                      tunnel: w308 -> [_ _]
                      tunnel: w307 -> [w312 _]
                      frame False {
                        # "Was Calculated."
                        # "calculated transform confirmed"
                        # "convert this to a modify"
                        n212 = Unbundle By Name(w312) -> ("X"=w315:dbl, "Y"=w314:dbl, "Z"=w313:dbl, "Notes"=w320:string)
                        n213 = local read "Notes:"() -> (w321:string)
                        n214 = Concatenate Strings(w320, w321) -> (w319:string)
                        n215 = local write "X-Position"(w315) -> ()
                        n216 = local write "Z-Position"(w313) -> ()
                        n217 = local write "Y-Position"(w314) -> ()
                        n218 = property on="Notes:" class="Str"("Val(Sgnl)"=w319) -> ()  [unwired: 2 in, 2 out]
                        n219 = local write "Group Coding"(12 ("Group Coding")) -> ()
                        n220 = Format Into String(format string="Enough fiducials have been entered to calculate the position\nof this spot. The calcuated position for this spot is:\nX = %f\nY = %f\nZ = %f \nThe value of the coordinates has been transfered to the\nAdd Spot Dialog box for you convenience.  You may correct\nthe position.", w315, w314, w313) -> (resulting string=w316:string)  [unwired: 2 in, 1 out]
                        n221 = One Button Dialog ("Drive to the Calculated Coordinates")(message=w316) -> ()  [unwired: 1 in, 1 out]
                      }
                      frame True {
                        w322 = 10 ("Original_group")
                        n222 = local write "Group Coding"(w322) -> ()
                        n223 = local write "Original_group"(w322) -> ()
                        n224 = One Button Dialog(message="The old point will be\nkept in the database\nof this session. You may\nstill press cancel to leave\nthe database as it was.") -> ()  [unwired: 1 in, 1 out]
                      }
                    }
                  }
                }
              }
              frame -1 {
                n225 = local read "Fiducial?"() -> (w325:bool)
                n226 = case shown="False" w325 {
                  tunnel: w324 -> [w327 _]
                  frame False {
                    n227 = local read "ArrayOfPointNames"() -> (w328:string[])
                    n228 = for {
                      tunnel: w328 -> [w332] mode=indexing
                      tunnel: w327 -> [w331]
                      tunnel: [w330] -> w326
                      stop <- w330 stop-if-true
                      n229 = Equal?(x=w332, y=w331) -> (x = y?=w330:bool)
                    }
                    n230 = case shown="True" w326 {
                      frame False {
                      }
                      frame True {
                        # "warn user that they are adding a pont that\nprobably could be transformed."
                        n231 = One Button Dialog(message="Warning: This position name exists in a previous\nsession. Normally you will want to transform\nfrom that session after you have found sufficinet\nfiducial. Press cancel if you do not want to add now.") -> ()  [unwired: 1 in, 1 out]
                      }
                    }
                  }
                  frame True {
                  }
                }
              }
              frame 0, 10, 12 {
                n232 = case shown="True" w335 {
                  tunnel: w334 -> [_ w340]
                  tunnel: w333 -> [_ _]
                  tunnel: w336 -> [_ w339]
                  frame False {
                  }
                  frame True {
                    # "if it is a calculated spot we want to\njust add that spot"
                    n233 = local read "Modify"() -> (w338:bool)
                    n234 = local read "Fiducial?"() -> (w337:bool)
                    n235 = case shown="False" w338 {
                      tunnel: w340 -> [w343 _]
                      tunnel: w337 -> [w342 _]
                      tunnel: w339 -> [w341 _]
                      frame False {
                        n236 = case shown="True" w342 {
                          tunnel: w343 -> [w346 _]
                          tunnel: w341 -> [_ w373]
                          frame False {
                            n237 = Random Number (0-1)() -> (number: 0 to 1=w354:dbl)
                            n238 = Multiply(x=w354, y=10000) -> (x*y=w350:dbl)
                            n239 = Round Toward -Infinity(1:w350) -> (0:w349:dbl)
                            n240 = To Unsigned Long Integer(number=w349) -> (unsigned 32bit integer=w348:u32)
                            n241 = Format Into String(w348) -> (resulting string=w351:string)  [unwired: 3 in, 1 out]
                            n242 = One Button Dialog(message="You have chosen a spot name that duplicates one in this session. \nA random number has been appended to it. to make it unique. \nIf you intended to modify an existing spot, cancel this dialog and select the spot in the current session tab drop down and press modify.") -> ()  [unwired: 1 in, 1 out]
                            n243 = Concatenate Strings(w346, "-" ("string"), w351) -> (w352:string)
                            n244 = property on="Point Name" class="Str"("Val(Sgnl)"=w352, "DisabledEnum"=T7."Enabled" ("Disabled")) -> ()  [unwired: 2 in, 2 out]
                          }
                          frame True {
                            n245 = local read "X-Position"() -> (w366:dbl)
                            n246 = Unbundle By Name(w373) -> ("OtherRelatedDataFiles"=w356:T6, "Notes"=w358:string, "Group"=w355:i32, "Rotation"=w360:dbl[unit], "Z"=w361:dbl, "X"=w367:dbl, "Y"=w370:dbl)
                            n247 = local read "Y-Position"() -> (w368:dbl)
                            n248 = local read "Notes:"() -> (w359:string)
                            n249 = Concatenate Strings(w358, w359) -> (w357:string)
                            n250 = Not A Number/Path/Refnum?(number/path/refnum=w366) -> (NaN/Path/Refnum?=w372:bool)
                            n251 = Not A Number/Path/Refnum?(number/path/refnum=w368) -> (NaN/Path/Refnum?=w371:bool)
                            n252 = Select(t=w367, s=w372, f=w366) -> (s? t:f=w365:dbl)
                            n253 = Select(t=w370, s=w371, f=w368) -> (s? t:f=w369:dbl)
                            n254 = local write "Z-Position"(w361) -> ()
                            n255 = node(w360) -> (w362:dbl)
                            n256 = local write "OtherRelatedDataFiles"(w356) -> ()
                            n257 = local write "Notes:"(w357) -> ()
                            n258 = local write "Original_group"(w355) -> ()
                            n259 = local write "StageRotation"(w362) -> ()
                            n260 = local write "X-Position"(w365) -> ()
                            n261 = local write "Y-Position"(w369) -> ()
                            n262 = property on="Move to next screen" class="Bool (strict)"("DisabledEnum"=T7."Disabled and Grayed Out" ("Disabled"), "TipStrip"="Coordinates need to be confirmed. Click in X or Y field\nand confirm the correct value to enable this button." ("Tip Strip")) -> ()  [unwired: 2 in, 2 out]
                            n263 = One Button Dialog(message="This fiducial has previously been\nentered. Program will assume\nyou want to make a correction.\nIf not select a different\nspot or press cancel. \nIf you had not entered coordinates\nfor this spot the old coords have been\nentered in X/Y positions fields.") -> ()  [unwired: 1 in, 1 out]
                          }
                        }
                      }
                      frame True {
                        # "Dont error on modify on spot name if\nthe  name is the same. It should be."
                      }
                    }
                  }
                }
              }
            }
          }
          event "Cancel Button": Value Change {
            n264 = event-data() -> ()  [unwired: 1 in, 5 out]
            n265 = local write "Cancel Button"(FALSE ("Cancel")) -> ()
            n266 = Two Button Dialog(message="You have selected cancel adding this spot to the DataBase. Press \"Yes\" if that's what you intended.", 1:"Don't Cancel this Spot" ("F button name (\"Cancel\")"), 2:"YES. do not save this spot" ("T button name (\"OK\")")) -> (T button?=w376:bool)
            n267 = local write "Cancel_OUT"(w376) -> ()
          }
          event "Add A Spot Related Data File": Value Change {
            # "prompt user for adding\na file"
            n268 = event-data() -> ()  [unwired: 1 in, 5 out]
            n269 = local read "OtherRelatedDataFiles"() -> (w382:T6)
            n270 = Array Size(array=w382) -> (size(s)=w381:i32)
            n271 = Greater Than 0?(x=w381) -> (x > 0?=w383:bool)
            n272 = case shown="False" w383 {
              tunnel: w382 -> [_ w391]
              tunnel: w381 -> [_ w393]
              tunnel: [path "" w389] -> w380
              frame False {
              }
              frame True {
                n273 = Decrement(x=w393) -> (x-1=w392:i32)
                n274 = Index Array(array=w391, index=w392) -> (element=w390:cluster{"Type of File":string, "FileName":path})
                n275 = Unbundle By Name(w390) -> ("FileName"=w389:path)
              }
            }
            n276 = call "Add_related_file.vi"("Path"=w380) -> ("Type or Description of File Out"=w385:string, "Path_out"=w386:path, "Cancelled?"=w387:bool)  [unwired: 8 in]
            n277 = case shown="False" w387 {
              tunnel: w386 -> [w398 _]
              tunnel: w385 -> [w397 _]
              tunnel: w382 -> [w394 _]
              frame False {
                n278 = Bundle By Name(cluster=cluster{"Type of File":string, "FileName":path} {"Type of File"="", "FileName"=path ""} ("element"), "FileName"=w398, "Type of File"=w397) -> (w396:cluster{"Type of File":string, "FileName":path})
                n279 = Build Array (concatenate)(w394, w396) -> (w395:T6)
                n280 = local write "OtherRelatedDataFiles"(w395) -> ()
              }
              frame True {
              }
            }
            n281 = local write "Add A Spot Related Data File"(FALSE ("Add A Spot Related Data File")) -> ()
          }
          event "Press to goto final Screen", "Tab Control": Value Change {
            w406 = 0.0 ("Magnification")
            # "new coding on group\n10 - is a user entered item"
            n282 = event-data() -> ("CtlRef"=w403:refnum<vi>)  [unwired: 1 in, 4 out]
            n283 = local read "X-Position"() -> (w415:dbl)
            n284 = local read "Y-Position"() -> (w416:dbl)
            n285 = local read "Z-Position"() -> (w414:dbl)
            n286 = local read "StageRotation"() -> (w413:dbl)
            n287 = local read "Group Coding"() -> (w405:i32)
            n288 = local read "MetaDataFile"() -> (w417:path)
            n289 = local read "Point Name"() -> (w408:string)
            n290 = property class="Ctl"(reference=w403) -> ("Label.Text"=w402:string)  [unwired: 1 in, 2 out]
            n291 = local read "Fiducial?"() -> (w411:bool)
            n292 = local read "Notes:"() -> (w409:string)
            n293 = local read "MetaDataAvailable"() -> (w410:bool)
            n294 = node(w413) -> (w412:dbl[unit])
            n295 = local read "OtherRelatedDataFiles"() -> (w407:T6)
            n296 = local read "PointInformation_IN"() -> (w404:T1)
            n297 = Equal?(x=w402, y="Press to goto final Screen") -> (x = y?=w400:bool)
            n298 = Bundle By Name(cluster=w404, "MetaDataFile"=w417, "X"=w415, "Y"=w416, "Group"=w405, "Z"=w414, "Rotation"=w412, "Fiducial"=w411, "Magnification"=w406, "Working_Distance"=w406, "Notes"=w409, "Location Name/ID"=w408, "OtherRelatedDataFiles"=w407, "Available"=w410) -> (w418:T1)
            n299 = case shown="True" w400 {
              frame False {
              }
              frame True {
                n300 = local write "Tab Control"(T4."SpotSummary" ("Tab Control")) -> ()
              }
            }
            n301 = local write "Press to goto final Screen"(FALSE ("Press to goto final Screen")) -> ()
            n302 = local write "Review Point Information"(w418) -> ()
          }
          event "Go Back to Correct": Value Change {
            n303 = event-data() -> ()  [unwired: 1 in, 5 out]
            n304 = local write "Go Back to Correct"(FALSE ("Go Back to Correct")) -> ()
            n305 = local write "Tab Control"(T4."Name and Postions" ("Tab Control")) -> ()
          }
          event "Notes:": Value Change {
            n306 = event-data() -> ("NewVal"=w423:string)  [unwired: 1 in, 4 out]
            n307 = local read "Review Point Information"() -> (w424:T1)
            n308 = Bundle By Name(cluster=w424, "Notes"=w423) -> (w425:T1)
            n309 = local write "Review Point Information"(w425) -> ()
          }
        }
      }
    }
  }
